vi "Handle_CoolpropData.vi"(11 "element":T3) -> (3 "output Array clusters":T1)   [LabVIEW 2022 SP3]
uses:
  TypeDefs/CoolPropArrayData.ctl
  Coolprop_64bit/CoolProp_advanced.llb/FluidCommon.ctl
  Coolprop_64bit/Coolprop_lib.lvlib
  TypeDefs/DataFraCoolProp.ctl
  TypeDefs/CoolPropArrays.ctl
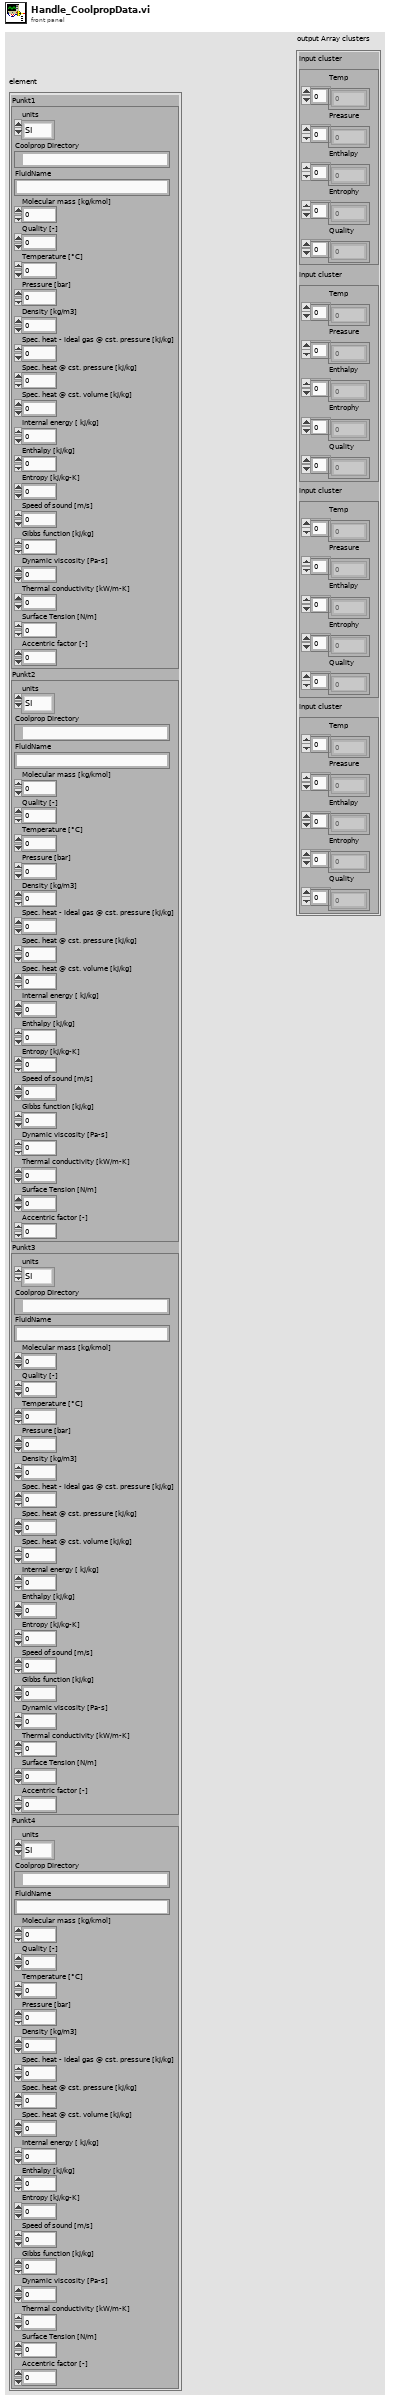
[diagram p1: front panel]
types:
  T1 = typedef "CoolPropArrays.ctl" = cluster{"input cluster":T2, "input cluster":T2, "input cluster":T2, "input cluster":T2}
  T2 = typedef "CoolPropArrayData.ctl" = cluster{"Temp":dbl[], "Preasure":dbl[], "Enthalpy":dbl[], "Entrophy":dbl[], "Quality":dbl[]}
  T3 = typedef "DataFraCoolProp.ctl" = cluster{"Punkt1":T4, "Punkt2":T4, "Punkt3":T4, "Punkt4":T4}
  T4 = typedef "Coolprop_lib.lvlib/FluidCommon.ctl" = cluster{"units":enum16{"SI", "IP"}, "Coolprop Directory":path, "FluidName":string, "Molecular mass [kg/kmol]":dbl, "Quality [-]":dbl, "Temperature [°C]":dbl, "Pressure [bar]":dbl, "Density [kg/m3]":dbl, "Spec. heat - ideal gas @ cst. pressure [kJ/kg]":dbl, "Spec. heat @ cst. pressure [kJ/kg]":dbl, "Spec. heat @ cst. volume [kJ/kg]":dbl, "Internal energy [ kJ/kg]":dbl, "Enthalpy [kJ/kg]":dbl, "Entropy [kJ/kg-K]":dbl, "Speed of sound [m/s]":dbl, "Gibbs function [kJ/kg]":dbl, "Dynamic viscosity [Pa-s]":dbl, "Thermal conductivity [kW/m-K]":dbl, "Surface Tension [N/m]":dbl, "Accentric factor [-]":dbl}
  T5 = cluster{"input cluster":T2, "input cluster":T2, "input cluster":T2, "input cluster":T2}
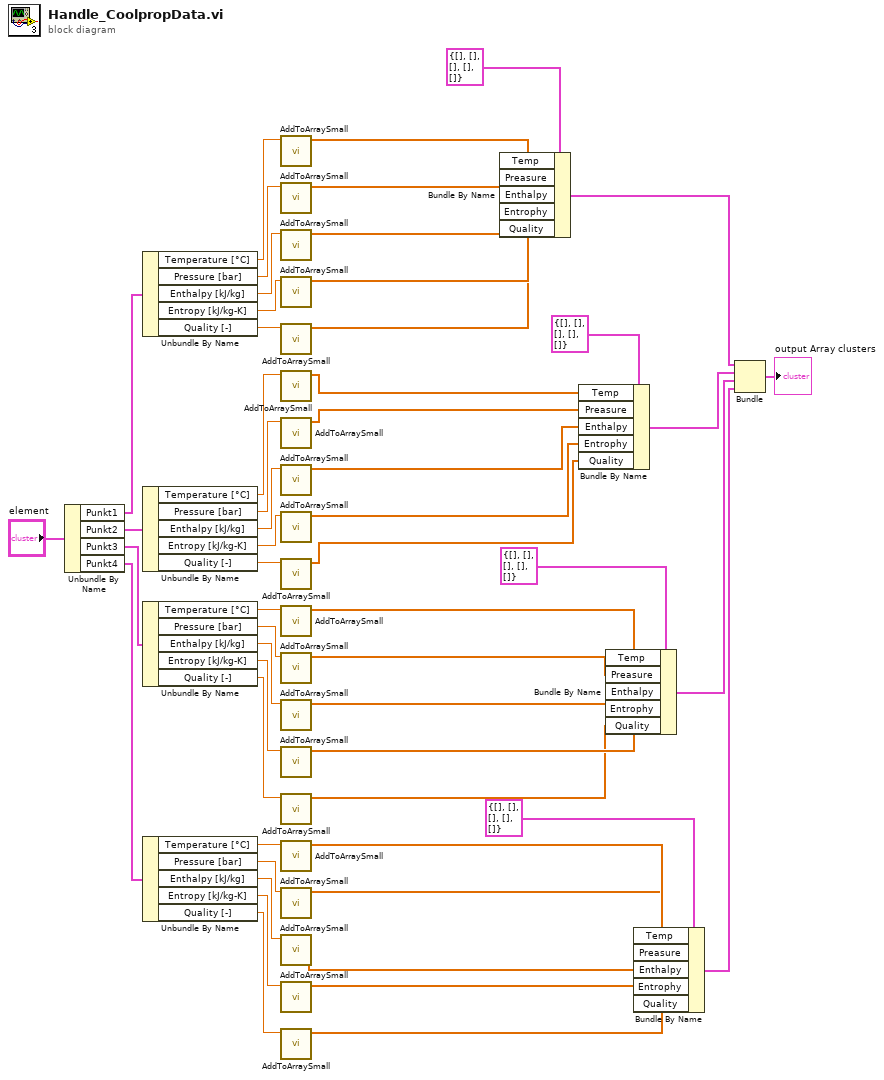
[diagram p0: block diagram]
diagram:
  n1 = Unbundle By Name("element") -> ("Punkt1"=w50:T4, "Punkt2"=w48:T4, "Punkt3"=w47:T4, "Punkt4"=w46:T4)
  n2 = Unbundle By Name(w50) -> ("Temperature [°C]"=w51:dbl, "Pressure [bar]"=w52:dbl, "Enthalpy [kJ/kg]"=w53:dbl, "Entropy [kJ/kg-K]"=w54:dbl, "Quality [-]"=w33:dbl)
  n3 = Unbundle By Name(w48) -> ("Temperature [°C]"=w45:dbl, "Pressure [bar]"=w44:dbl, "Enthalpy [kJ/kg]"=w43:dbl, "Entropy [kJ/kg-K]"=w42:dbl, "Quality [-]"=w32:dbl)
  n4 = Unbundle By Name(w47) -> ("Temperature [°C]"=w41:dbl, "Pressure [bar]"=w40:dbl, "Enthalpy [kJ/kg]"=w39:dbl, "Entropy [kJ/kg-K]"=w38:dbl, "Quality [-]"=w31:dbl)
  n5 = Unbundle By Name(w46) -> ("Temperature [°C]"=w37:dbl, "Pressure [bar]"=w36:dbl, "Enthalpy [kJ/kg]"=w35:dbl, "Entropy [kJ/kg-K]"=w34:dbl, "Quality [-]"=w30:dbl)
  n6 = call "AddToArraySmall.vi"("Input"=w51) -> ("output array"=w29:dbl[])  [unwired: 10 in]
  n7 = call "AddToArraySmall.vi"("Input"=w52) -> ("output array"=w28:dbl[])  [unwired: 10 in]
  n8 = call "AddToArraySmall.vi"("Input"=w53) -> ("output array"=w27:dbl[])  [unwired: 10 in]
  n9 = call "AddToArraySmall.vi"("Input"=w54) -> ("output array"=w26:dbl[])  [unwired: 10 in]
  n10 = call "AddToArraySmall.vi"("Input"=w33) -> ("output array"=w25:dbl[])  [unwired: 10 in]
  n11 = call "AddToArraySmall.vi"("Input"=w45) -> ("output array"=w20:dbl[])  [unwired: 10 in]
  n12 = call "AddToArraySmall.vi"("Input"=w44) -> ("output array"=w19:dbl[])  [unwired: 10 in]
  n13 = call "AddToArraySmall.vi"("Input"=w43) -> ("output array"=w18:dbl[])  [unwired: 10 in]
  n14 = call "AddToArraySmall.vi"("Input"=w42) -> ("output array"=w17:dbl[])  [unwired: 10 in]
  n15 = call "AddToArraySmall.vi"("Input"=w32) -> ("output array"=w16:dbl[])  [unwired: 10 in]
  n16 = call "AddToArraySmall.vi"("Input"=w41) -> ("output array"=w15:dbl[])  [unwired: 10 in]
  n17 = call "AddToArraySmall.vi"("Input"=w40) -> ("output array"=w14:dbl[])  [unwired: 10 in]
  n18 = call "AddToArraySmall.vi"("Input"=w39) -> ("output array"=w13:dbl[])  [unwired: 10 in]
  n19 = call "AddToArraySmall.vi"("Input"=w38) -> ("output array"=w12:dbl[])  [unwired: 10 in]
  n20 = call "AddToArraySmall.vi"("Input"=w31) -> ("output array"=w11:dbl[])  [unwired: 10 in]
  n21 = call "AddToArraySmall.vi"("Input"=w37) -> ("output array"=w10:dbl[])  [unwired: 10 in]
  n22 = call "AddToArraySmall.vi"("Input"=w36) -> ("output array"=w9:dbl[])  [unwired: 10 in]
  n23 = call "AddToArraySmall.vi"("Input"=w35) -> ("output array"=w8:dbl[])  [unwired: 10 in]
  n24 = call "AddToArraySmall.vi"("Input"=w34) -> ("output array"=w7:dbl[])  [unwired: 10 in]
  n25 = call "AddToArraySmall.vi"("Input"=w30) -> ("output array"=w6:dbl[])  [unwired: 10 in]
  n26 = Bundle By Name(cluster=T2 {"Temp"=[], "Preasure"=[], "Enthalpy"=[], "Entrophy"=[], "Quality"=[]} ("input cluster"), "Temp"=w29, "Preasure"=w28, "Enthalpy"=w27, "Entrophy"=w26, "Quality"=w25) -> (w5:T2)
  n27 = Bundle By Name(cluster=T2 {"Temp"=[], "Preasure"=[], "Enthalpy"=[], "Entrophy"=[], "Quality"=[]} ("input cluster"), "Temp"=w20, "Preasure"=w19, "Enthalpy"=w18, "Entrophy"=w17, "Quality"=w16) -> (w4:T2)
  n28 = Bundle By Name(cluster=T2 {"Temp"=[], "Preasure"=[], "Enthalpy"=[], "Entrophy"=[], "Quality"=[]} ("input cluster"), "Temp"=w15, "Preasure"=w14, "Enthalpy"=w13, "Entrophy"=w12, "Quality"=w11) -> (w3:T2)
  n29 = Bundle By Name(cluster=T2 {"Temp"=[], "Preasure"=[], "Enthalpy"=[], "Entrophy"=[], "Quality"=[]} ("input cluster"), "Temp"=w10, "Preasure"=w9, "Enthalpy"=w8, "Entrophy"=w7, "Quality"=w6) -> (w2:T2)
  n30 = Bundle("input cluster"=w5, "input cluster"=w4, "input cluster"=w3, "input cluster"=w2) -> (→"output Array clusters":T5)  [unwired: 1 in]
